vi "Drive Path.vi"(5 "Timeout ms (-1)":i32=-1, 7 "Wait for Completion? (F)":bool, 8 "error in":errorcluster, 9 "Force? (F)":bool, 10 "Right":T1[](array[typedef]), 11 "Left":T1[](array[typedef])) -> (0 "error out":errorcluster)   [LabVIEW 2016, in "Drive System.lvlib"]
uses:
  Drive System.lvlib
  Pathfinder/VIs/Segment.ctl
  Private/DriveCmd.ctl
  Private/DriveCmdList.ctl
  Private/Varient Cmd Types/Follow Path.ctl
  Pathfinder/Pathfinder.lvlib
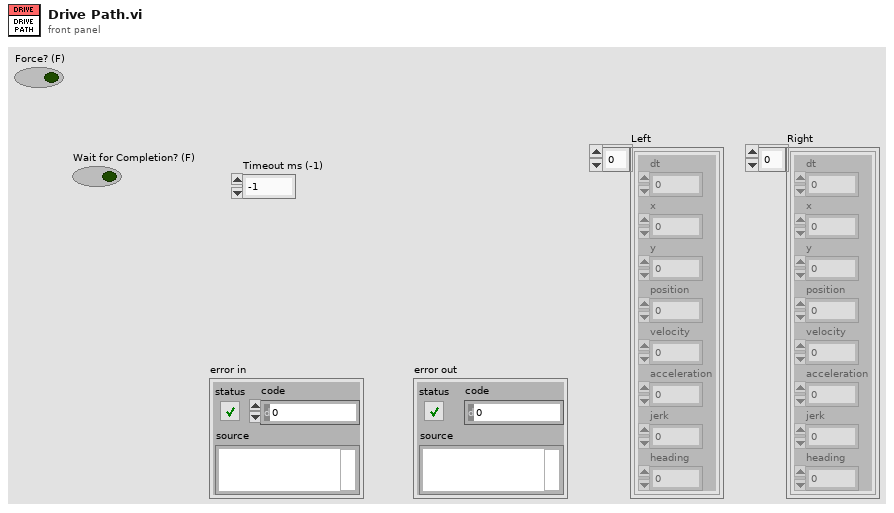
[diagram p1: front panel]
types:
  T1 = typedef "Pathfinder.lvlib/Segment.ctl" = cluster{"dt":dbl, "x":dbl, "y":dbl, "position":dbl, "velocity":dbl, "acceleration":dbl, "jerk":dbl, "heading":dbl}
  T2 = typedef "Drive System.lvlib/Follow Path.ctl" = cluster{"Left":T1[], "Right":T1[]}
  T3 = typedef "Drive System.lvlib/DriveCmd.ctl" = cluster{"cmd":T4, "data":variant, "Force? (F)":bool, "Lock":string}
  T4 = typedef "Drive System.lvlib/DriveCmdList.ctl" = enum16{"Idle", "Cleanup", "Drive For Time", "Follow Path", "Drive Tank", "Drive Arcade", "Unlock", "Lock"}
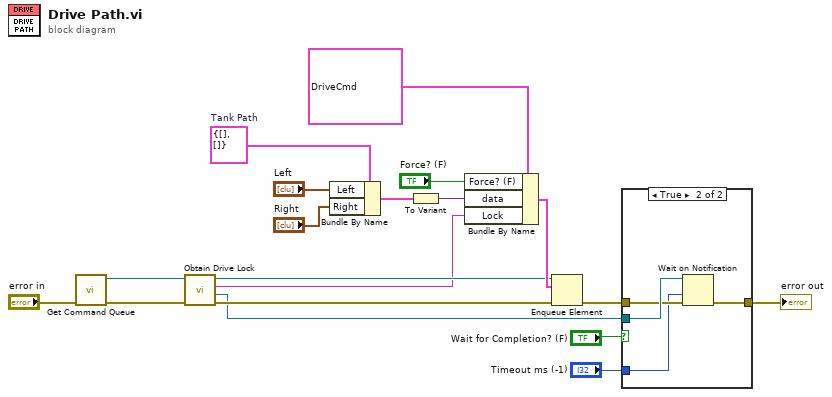
[diagram p0: block diagram]
diagram:
  w8 = T2 {"Left"=[], "Right"=[]}  # Tank Path
  n1 = call "Get Command Queue.vi"("error in (no error)"="error in") -> ("error out"=w19:errorcluster, "Queue out"=w18:refnum<queue>)  [unwired: 9 in]
  n2 = call "Obtain Drive Lock.vi"("error in"=w19, "Queue in"=w18) -> ("error out"=w11:errorcluster, "notifier out"=w3:refnum<notifier>, "Lock"=w9:string, "queue out"=w10:refnum<queue>)  [unwired: 6 in]
  n3 = Bundle By Name(cluster=w8, "Left"="Left", "Right"="Right") -> (w14:T2)
  n4 = To Variant(anything=w14) -> (Variant=w15:variant)
  n5 = Bundle By Name(cluster=T3 {"cmd"=enum."Follow Path", "data"=variant, "Force? (F)"=FALSE, "Lock"=""} ("element"), "Force? (F)"="Force? (F)", "data"=w15, "Lock"=w9) -> (w16:T3)
  n6 = Enqueue Element(queue=w10, element=w16, error in (no error)=w11) -> (error out=w5:errorcluster)  [unwired: 1 in, 2 out]
  n7 = case shown="True" "Wait for Completion? (F)" {
    tunnel: w5 -> [w20 w23]
    tunnel: w3 -> [_ w24]
    tunnel: [w20 w22] -> w4
    tunnel: "Timeout ms (-1)" -> [_ w21]
    frame False {
    }
    frame True {
      n8 = Wait on Notification(notifier=w24, timeout in ms (-1)=w21, error in (no error)=w23) -> (error out=w22:errorcluster)  [unwired: 1 in, 3 out]
    }
  }
  "error out" <- w4
